vi "移位寄存器3vi.vi"() -> ()   [LabVIEW 2023]
panel:
  out "输出寄存 3":i32
  out "输入寄存 2":i32
  out "输入寄存":i32
  out "输入寄存 3":i32
  out "输出寄存 2":i32
  out "输出寄存":i32
  out "输出寄存器":i32
  out "输入寄存器":i32
  # "移位寄存器 3"
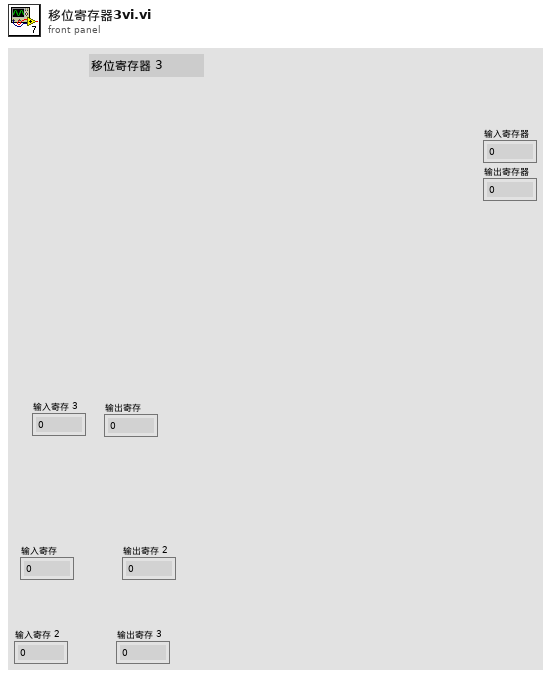
[diagram p1: front panel]
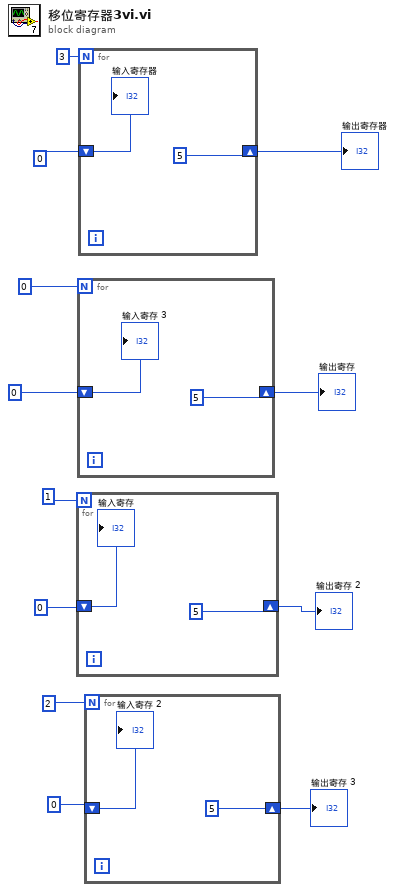
[diagram p0: block diagram]
diagram:
  n1 = for {
    N: 1 -> [_]
    shift-right: [5] -> w4
    shift-left: 0 -> [w13]
    "输入寄存" <- w13
  }
  "输出寄存 2" <- w4
  n2 = for {
    N: 0 -> [_]
    shift-right: [5] -> w7
    shift-left: 0 -> [w15]
    "输入寄存 3" <- w15
  }
  "输出寄存" <- w7
  n3 = for {
    N: 3 -> [_]
    shift-right: [5] -> w10
    shift-left: 0 -> [w17]
    "输入寄存器" <- w17
  }
  "输出寄存器" <- w10
  n4 = for {
    N: 2 -> [_]
    shift-right: [5] -> w1
    shift-left: 0 -> [w19]
    "输入寄存 2" <- w19
  }
  "输出寄存 3" <- w1
